vi "Window-Combo box editor.vi"(11 "Combo box ref":refnum<vi>) -> (1 "Cancelled":bool)   [LabVIEW 2017]
uses:
  Global Variables/General Globals.vi
panel:
  out "Initial values":string[](array[string])
  in  "Apply & Exit":bool
  in  "Values":string[](array[string])
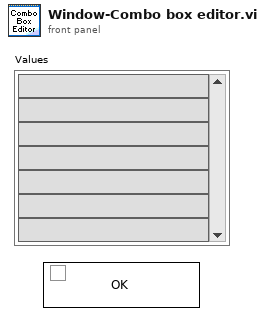
[diagram p1: front panel]
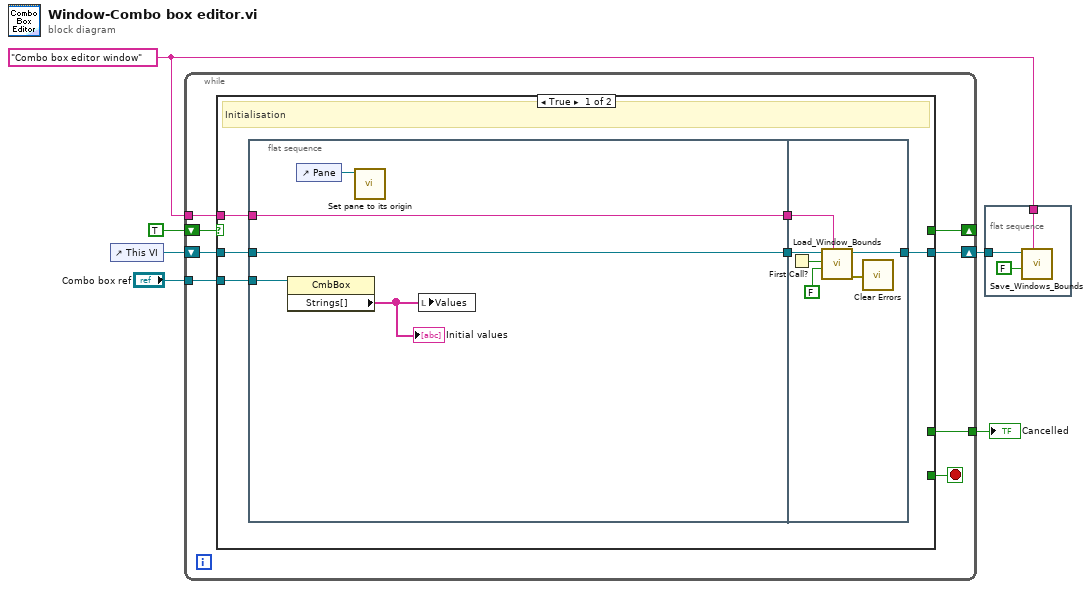
[diagram p0: block diagram]
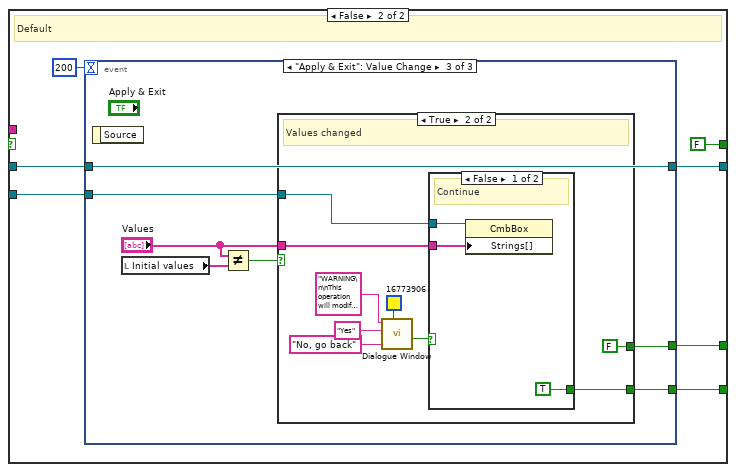
[diagram p2: hidden frame]
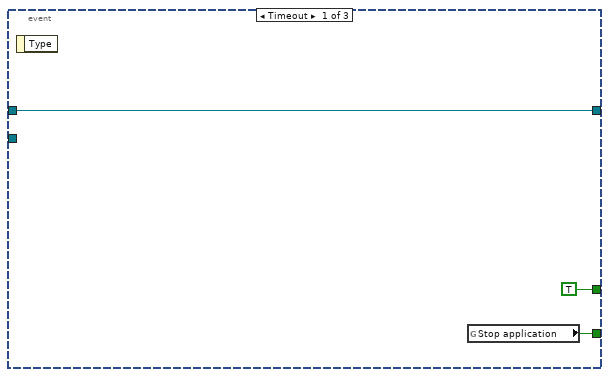
[diagram p3: hidden frame]
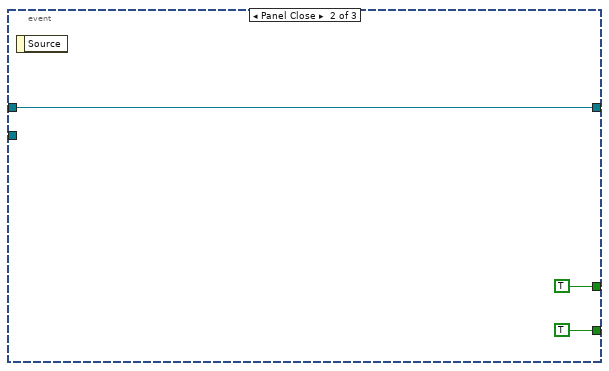
[diagram p4: hidden frame]
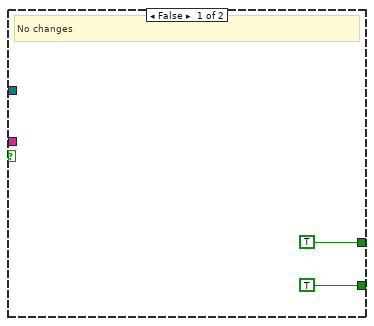
[diagram p5: hidden frame]
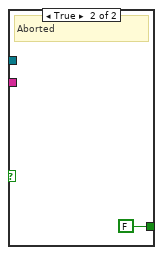
[diagram p6: hidden frame]
diagram:
  w3 = "Combo box editor window" ("Window Name (i.e. Key)")
  n1 = control-ref of="This VI"() -> (w6:refnum<vi>)
  n2 = while {
    shift-right: [w9] -> _
    shift-left: TRUE -> [w10]
    shift-right: [w13] -> w4
    shift-left: w6 -> [w12]
    tunnel: w3 -> [w11]
    tunnel: "Combo box ref" -> [w8]
    tunnel: [w7] -> w2
    stop <- w14 stop-if-true
    n3 = case shown="True" w10 {
      tunnel: [_ w38] -> w14
      tunnel: [w16 w37] -> w13
      tunnel: w12 -> [w17 w36]
      tunnel: w11 -> [w18 _]
      tunnel: [_ FALSE] -> w9
      tunnel: w8 -> [w15 w32]
      tunnel: [_ w33] -> w7
      frame True {
        # "Initialisation"
        n4 = flat-sequence {
          tunnel: w17 -> [w25]
          tunnel: [w25] -> w20
          tunnel: [w24] -> w19
          tunnel: w18 -> [w24]
          tunnel: w15 -> [w23]
          tunnel: [w30] -> w16
          tunnel: w20 -> [w31]
          tunnel: w19 -> [w28]
          frame #0 {
            n5 = property class="CmbBox"(reference=w23) -> ("Strings[]"=w21:string[])  [unwired: 1 in, 2 out]
            "Initial values" <- w21
            n6 = control-ref of="Pane"() -> (w22:refnum<vi>)
            n7 = call <userlib>:"Set pane to its origin.vi"("Pane Reference"=w22) -> ()  [unwired: 9 in, 2 out]
            n8 = local write "Values"(w21) -> ()
          }
          frame #1 {
            n9 = First Call?() -> (First Call?: T/F=w27:bool)
            n10 = call "Load_Window_Bounds.vi"("Window Name (i.e. Key)"=w28, "Disable"=FALSE, "First Call"=w27, "Window VI's Ref"=w31) -> ("error out"=w29:errorcluster, "reference out"=w30:refnum<vi>)  [unwired: 4 in, 2 out]
            n11 = call <vilib>:"Clear Errors.vi"("error in (no error)"=w29) -> ()  [unwired: 5 in, 2 out]
          }
        }
      }
      frame False {
        # "Default"
        n12 = event shown="[2] \"Apply & Exit\": Value Change" {
          selector: _ -> [_ _ _]
          dyn-events: _ -> [_ _ _]
          timeout: 200 -> [_ _ _]
          tunnel: [w39 TRUE ("Main Parallel Loop") w50] -> w38
          tunnel: [w41 w43 w51] -> w37
          tunnel: w36 -> [w41 w43 w51]
          tunnel: [TRUE ("Main Parallel Loop") TRUE ("Main Parallel Loop") w45] -> w33
          tunnel: w32 -> [_ _ w47]
          event Timeout {
            n13 = event-data() -> ()  [unwired: 1 in, 1 out]
            n14 = global read "General Globals.vi" "Stop application"() -> (w39:bool)
          }
          event Panel Close {
            n15 = event-data() -> ()  [unwired: 1 in, 1 out]
          }
          event "Apply & Exit": Value Change {
            n16 = event-data() -> ()  [unwired: 1 in, 1 out]
            n17 = local read "Initial values"() -> (w48:string[])
            n18 = Not Equal?(x="Values", y=w48) -> (x != y?=w46:bool)
            n19 = case shown="True" w46 {
              tunnel: [TRUE ("Main Parallel Loop") w58] -> w50
              tunnel: "Values" -> [_ w57]
              tunnel: w47 -> [_ w56]
              tunnel: [TRUE ("Main Parallel Loop") FALSE ("Main Parallel Loop")] -> w45
              frame False {
                # "No changes"
              }
              frame True {
                # "Values changed"
                n20 = call "Dialogue Window.vi"("Colour"=u32 16773906, "Caption-Left button (Cancel)"="No, go back", "Caption-Right button (OK)"="Yes", "Message string"="WARNING\n\nThis operation will modify the hardware setup.\nAre you sure you want to do this?") -> ("Cancelled (Left button pressed)"=w59:bool)  [unwired: 5 in, 2 out]
                n21 = case shown="False" w59 {
                  tunnel: w57 -> [w65 _]
                  tunnel: w56 -> [w64 _]
                  tunnel: [TRUE ("Main Parallel Loop") FALSE ("Main Parallel Loop")] -> w58
                  frame False {
                    # "Continue"
                    n22 = property class="CmbBox"(reference=w64, "Strings[]"=w65) -> ()  [unwired: 1 in, 2 out]
                  }
                  frame True {
                    # "Aborted"
                  }
                }
              }
            }
          }
        }
      }
    }
  }
  "Cancelled" <- w2
  n23 = flat-sequence {
    tunnel: w4 -> [w69]
    tunnel: w3 -> [w67]
    frame #0 {
      n24 = call "Save_Windows_Bounds.vi"("Window Name (i.e. Key)"=w67, "Front Panel Window:Open"=FALSE, "Window VI's Ref"=w69) -> ()  [unwired: 8 in, 1 out]
    }
  }
